vi "Read Instruments.vi"(8 "error in (no error)":errorcluster, 11 "Manual UI in":refnum<class "Manual UI.lvclass">) -> (0 "error out":errorcluster, 2 "Instruments":T1(array[cluster]), 3 "Manual UI out":refnum<class "Manual UI.lvclass">)   [LabVIEW 2023, in "Manual UI.lvlib" / "Manual UI.lvclass"]
uses:
  Project/Manual UI.lvclass
  builds/Instruments/Instruments.lvlibp/Library/Instruments.lvclass
  Project/Manual UI.lvclass/Manual UI.ctl
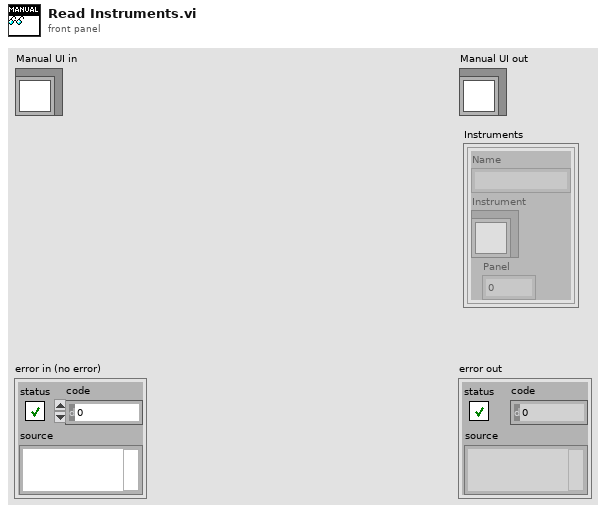
[diagram p1: front panel]
types:
  T1 = cluster{"Name":string, "Instrument":refnum<class "Instruments.lvclass">, "Panel":i32}[]
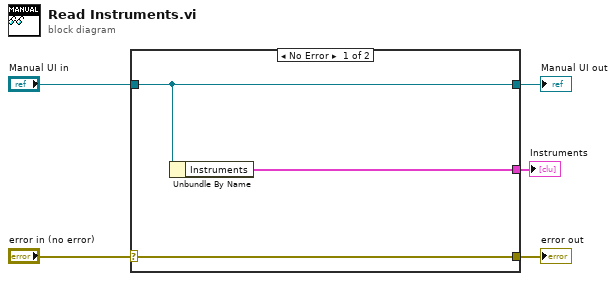
[diagram p0: block diagram]
diagram:
  n1 = case shown="No Error" "error in (no error)" {
    selector: "error in (no error)" -> [w8 w9]
    tunnel: [w8 w9] -> w4
    tunnel: [w7 w10] -> w2
    tunnel: "Manual UI in" -> [w7 w10]
    tunnel: [w6 _] -> w1
    frame No Error {
      n2 = Unbundle By Name(w7) -> ("Instruments"=w6:T1)
    }
    frame Error {
    }
  }
  "error out" <- w4
  "Manual UI out" <- w2
  "Instruments" <- w1
